vi "test_DL950_temperture.vi"() -> ()   [LabVIEW 2019]
uses:
  76b787d9-b2a3-4b08-af22-58dfa6f6235b.vi
  <instrlib>/Yokogawa DL950 Series/Public/Configure/Configure Module (Voltage).vi
  <instrlib>/Yokogawa DL950 Series/Public/Configure/Configure Module (Temperature).vi
  <instrlib>/Yokogawa DL950 Series/Yokogawa DL950 Series.lvlib
  f7627c64-1743-497c-a0ce-b64357051876.vi
panel:
  out "Waveform Data":waveform(dbl)[](graph)
  in  "Boolean 2":bool
  out "Array":dbl[](array[numeric])
  out "Waveform Chart":T1(graph)
  in  "write buffer":string=":CHANnel3:TEMPerature?"
  out "read buffer":string
  in  "Boolean":bool
  out "time":u32
  in  "정지":bool
  out "error out":errorcluster
  in  "visa":refnum<visa-resource-name>
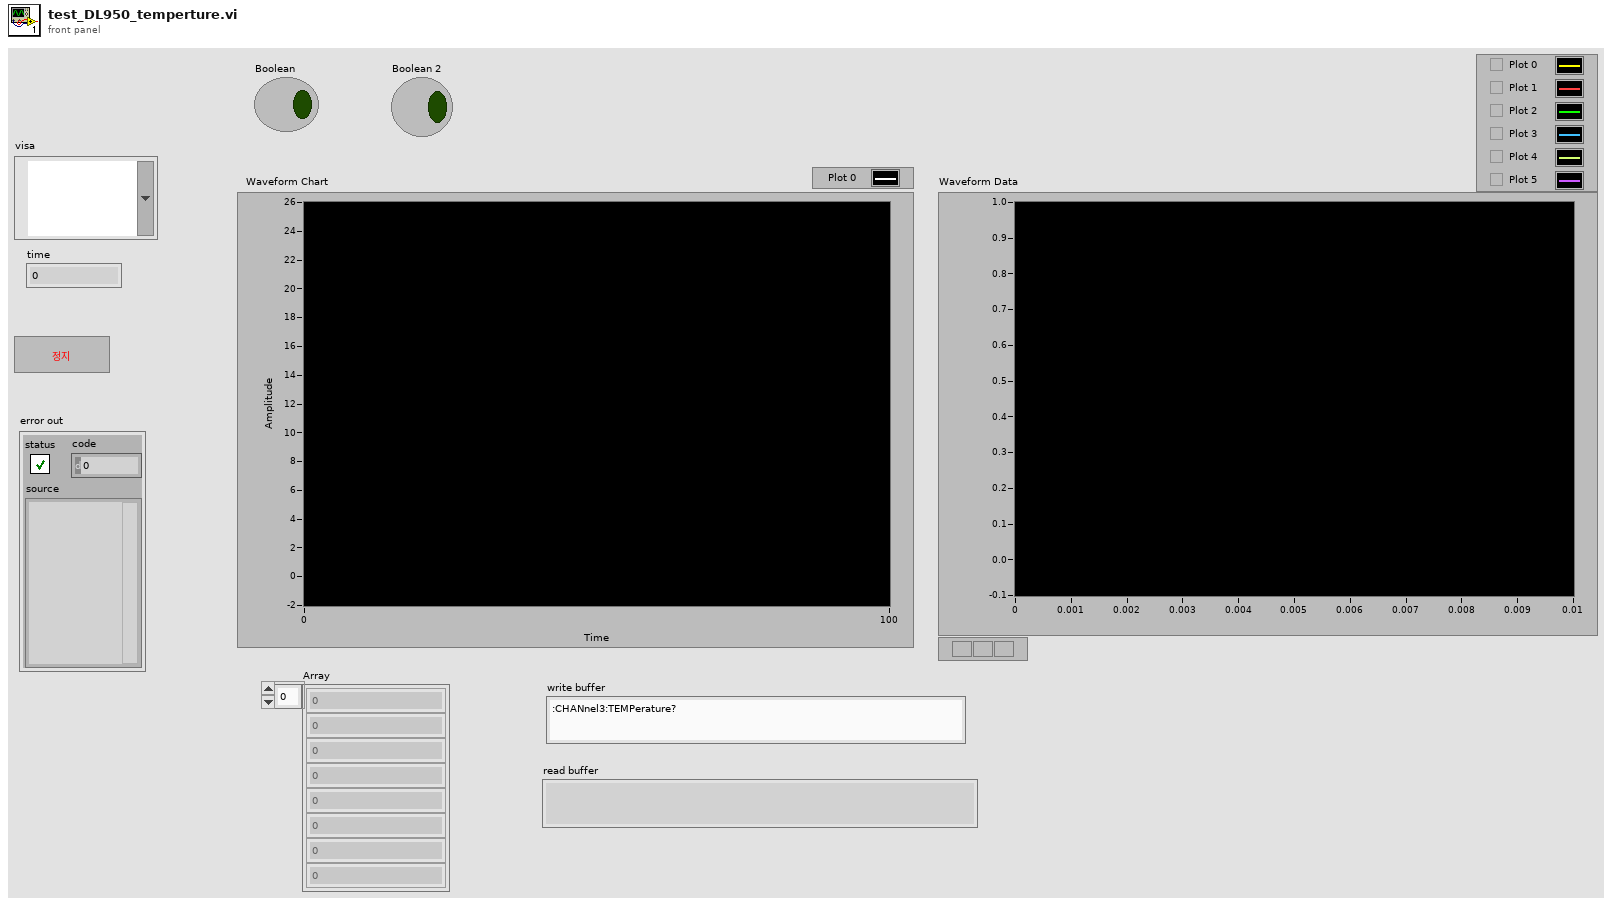
[diagram p1: front panel]
types:
  T1 = cluster{"[0]":dbl, "[1]":dbl, "[2]":dbl, "[3]":dbl, "[4]":dbl, "[5]":dbl, "[6]":dbl, "[7]":dbl, "[8]":dbl}
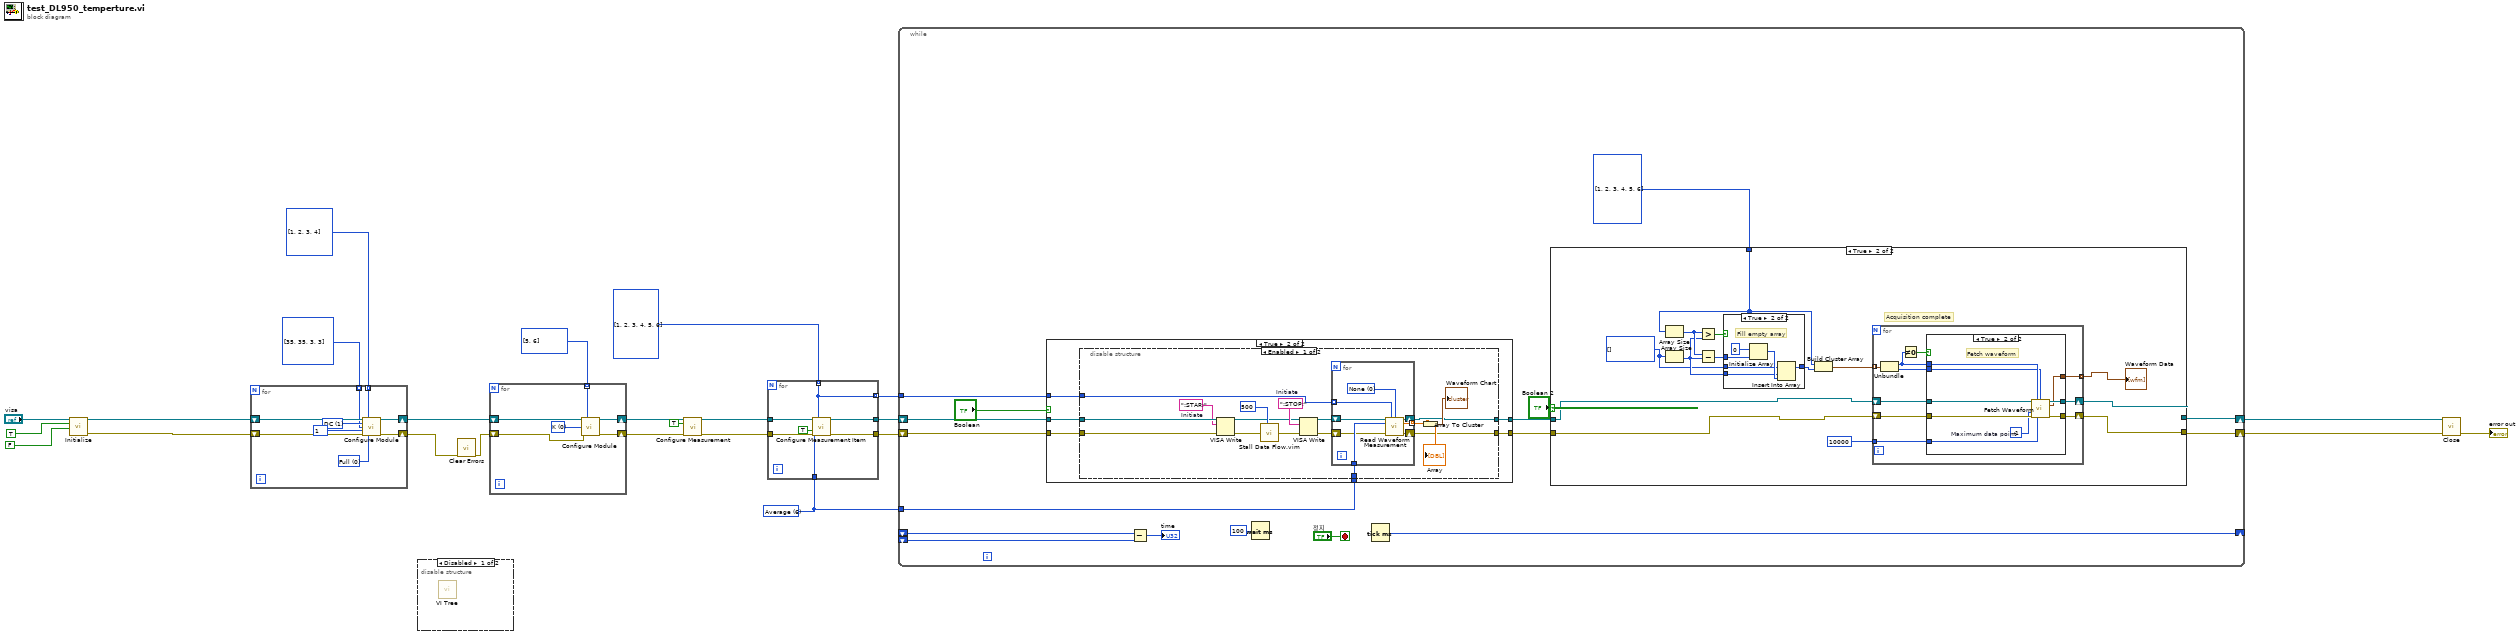
[diagram p0: block diagram]
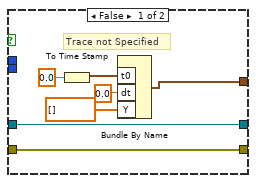
[diagram p4: hidden frame]
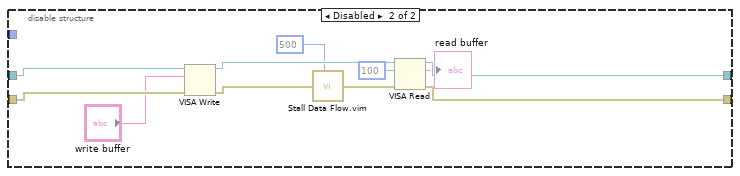
[diagram p7: hidden frame]
diagram:
  w8 = i32[] [35, 35, 3, 3] items=["1:1", "2:1", "5:1", "10:1", "20:1", "50:1", "100:1", "200:1", "500:1", "1000:1", "2000:1", "5000:1", "10k:1", "20k:1", "50k:1", "0.1A:1V", "0.2A:1V", "0.5A:1V", "1A:1V", "2A:1V", "5A:1V", "10A:1V", "20A:1V", "50A:1V", "100A:1V", "200A:1V", "250A:1V", "400A:1V", "500A:1V", "1kA:1V", "2kA:1V", "5kA:1V", "10kA:1V", "20kA:1V", "50kA:1V", "NoSet"]
  w9 = u16[] [1, 2, 3, 4] items=["", "CH1", "CH2", "CH3", "CH4", "CH5", "CH6", "CH7", "CH8", "CH9", "CH10", "CH11", "CH12", "CH13", "CH14", "CH15", "CH16"]
  w12 = u16[] [5, 6] items=["", "CH1", "CH2", "CH3", "CH4", "CH5", "CH6", "CH7", "CH8", "CH9", "CH10", "CH11", "CH12", "CH13", "CH14", "CH15", "CH16"]
  w13 = i32[] [1, 2, 3, 4, 5, 6] items=["", "CH1", "CH2", "CH3", "CH4", "CH5", "CH6", "CH7", "CH8", "CH9", "CH10", "CH11", "CH12", "CH13", "CH14", "CH15", "CH16", "RMATH1", "RMATH2", "RMATH3", "RMATH4", "RMATH5", "RMATH6", "RMATH7", "RMATH8", "RMATH9", "RMATH10", "RMATH11", "RMATH12", "RMATH13", "RMATH14", "RMATH15", "RMATH16", "MATH1", "MATH2", "MATH3", "MATH4", "MATH5", "MATH6", "MATH7", "MATH8"]
  w16 = 6 items=["Peak to Peak", "Amplitude", "Max", "Min", "High", "Low", "Average", "Middle", "Rms", "Standard Deviation", "+Overshoot", "-Overshoot", "Rise", "Fall", "Frequency", "Period", "+Width", "-Width", "Duty Cycle", "Pulse Count", "Burst1 Width", "Burst2 Width", "Average Frequency", "Average Period", "Int1TY", "Int2TY"] ("Measurement Item (0: Peak to Peak)")
  n1 = call <instrlib>:"Initialize.vi"("Reset (True)"=FALSE, "ID Query (True)"=TRUE, "VISA resource name"="visa") -> ("error out"=w1:errorcluster, "VISA resource name out"=w2:refnum<visa-resource-name>)  [unwired: 7 in]
  n2 = for {
    shift-right: [w31] -> w14
    shift-left: w2 -> [w33]
    shift-right: [w30] -> w11
    shift-left: w1 -> [w32]
    tunnel: w9 -> [w26] mode=indexing
    tunnel: w8 -> [w25] mode=indexing
    w28 = 12 items=["0.1m", "0.2m", "0.5m", "1m", "2m", "5m", "10m", "20m", "50m", "100m", "200m", "500m", "1", "2", "4", "5", "8", "10", "20", "40", "50", "80", "100", "200", "400", "500", "800", "1k", "2k", "4k", "5k", "8k", "10k", "20k", "25k", "50k", "100k", "250k", "500k", "1000k"] ("Vertical Division (20: 50)")
    w27 = 0 items=["Full", "Auto", "0.1Hz", "1Hz", "2Hz", "8Hz", "30Hz", "40Hz", "400Hz", "500Hz", "4kHz", "5kHz", "10kHz", "20kHz", "40kHz", "50kHz", "80kHz", "160kHz", "320kHz", "400kHz", "500kHz", "640kHz", "1.28MHz", "2MHz", "2.56MHz", "5MHz"] ("Bandwidth (0: Full)")
    w29 = 1 items=["AC", "DC", "Ground", "AC-RMS", "DC-RMS"] ("Vertical Coupling (1: DC)")
    n3 = call-poly <instrlib>:"Configure Module.vi"("VISA resource name"=w33, "Channel (1: CH1)"=w26, "Vertical Coupling (1: DC)"=w29, "Probe Attenuation (3: 10:1)"=w25, "Vertical Division (20: 50)"=w28, "error in (no error)"=w32, "Bandwidth (0: Full)"=w27) -> ("VISA resource name out"=w31:refnum<visa-resource-name>, "error out"=w30:errorcluster)  [unwired: 7 in]
  }
  n4 = disable-structure shown="Disabled" {
    frame Disabled {
      n5 = call <instrlib>:"VI Tree.vi"() -> ()  [unwired: 12 in]
    }
    frame Enabled {
    }
  }
  n6 = call <vilib>:"Clear Errors.vi"("error in (no error)"=w11) -> ("error out"=w10:errorcluster)  [unwired: 5 in, 1 out]
  n7 = for {
    shift-right: [w35] -> w5
    shift-left: w10 -> [w38]
    shift-right: [w36] -> w7
    shift-left: w14 -> [w37]
    tunnel: w12 -> [w34] mode=indexing
    w39 = 0 items=["K", "E", "J", "T", "L", "U", "N", "R", "S", "B", "W", "Au7fe"] ("Thermocouple Type (0: K)")
    n8 = call-poly <instrlib>:"Configure Module.vi"("VISA resource name"=w37, "Channel (1: CH1)"=w34, "Thermocouple Type (0: K)"=w39, "error in (no error)"=w38) -> ("VISA resource name out"=w36:refnum<visa-resource-name>, "error out"=w35:errorcluster)  [unwired: 10 in]
  }
  n9 = call <instrlib>:"Configure Measurement.vi"("VISA resource name"=w7, "Enable Measurement (True)"=TRUE, "error in (no error)"=w5) -> ("VISA resource name out"=w6:refnum<visa-resource-name>, "error out"=w4:errorcluster)  [unwired: 11 in]
  n10 = for {
    tunnel: [w46] -> w18
    tunnel: [w45] -> w17
    tunnel: w16 -> [w43]
    tunnel: [w40] -> w15 mode=indexing
    tunnel: w6 -> [w42]
    tunnel: w4 -> [w41]
    tunnel: w13 -> [w40] mode=indexing
    n11 = call <instrlib>:"Configure Measurement Item.vi"("VISA resource name"=w42, "Source (1: CH1)"=w40, "Measurement Item (0: Peak to Peak)"=w43, "Enable Measurement Item (False)"=TRUE, "error in (no error)"=w41) -> ("VISA resource name out"=w46:refnum<visa-resource-name>, "error out"=w45:errorcluster)  [unwired: 9 in]
  }
  n12 = while {
    shift-right: [w49] -> w20
    shift-left: w18 -> [w58]
    shift-right: [w48] -> w19
    shift-left: w17 -> [w57]
    shift-right: [w62] -> _
    shift-left: _ -> [w61]
    shift-left: _ -> [w60]
    tunnel: w16 -> [w56]
    tunnel: w15 -> [w53]
    stop <- "정지" stop-if-true
    w47 = u16[] [1, 2, 3, 4, 5, 6] items=["None", "CH1", "CH2", "CH3", "CH4", "CH5", "CH6", "CH7", "CH8", "CH9", "CH10", "CH11", "CH12", "CH13", "CH14", "CH15", "CH16", "MATH1", "MATH2", "MATH3", "MATH4", "MATH5", "MATH6", "MATH7", "MATH8", "EVENT"] ("Source (1: CH1)")
    n13 = case shown="True" "Boolean" {
      tunnel: w58 -> [w114 w120]
      tunnel: w57 -> [w113 w119]
      tunnel: [w114 w118] -> w51
      tunnel: [w113 w117] -> w50
      tunnel: w56 -> [_ w116]
      tunnel: w53 -> [_ w115]
      frame False {
      }
      frame True {
        n14 = disable-structure shown="Enabled" {
          disable-tunnel: w120 -> [w136 w155]
          disable-tunnel: w119 -> [w135 w154]
          disable-tunnel: [w122 w151] -> w118
          disable-tunnel: [w121 w150] -> w117
          disable-tunnel: w116 -> [w134 _]
          disable-tunnel: w115 -> [w125 _]
          frame Enabled {
            w130 = ":STOP;"  # Initiate
            w131 = ":STAR;"  # Initiate
            n15 = VISA Write ("VISA書き込み")(VISA resource name=w136, write buffer=w131, error in (no error)=w135) -> (VISA resource name out=w126:refnum<visa-resource-name>, error out=w129:errorcluster)  [unwired: 1 out]
            n16 = call "Stall Data Flow.vim"("value in"=w129, "milliseconds to wait"=u32 500 ("dt")) -> ("value out"=w128:errorcluster)  [unwired: 1 out]
            n17 = VISA Write ("VISA書き込み")(VISA resource name=w126, write buffer=w130, error in (no error)=w128) -> (VISA resource name out=w133:refnum<visa-resource-name>, error out=w132:errorcluster)  [unwired: 1 out]
            n18 = for {
              tunnel: w134 -> [w142]
              tunnel: [w138] -> w124 mode=indexing
              tunnel: w125 -> [w137] mode=indexing
              shift-right: [w144] -> w122
              shift-left: w133 -> [w140]
              shift-right: [w143] -> w121
              shift-left: w132 -> [w139]
              w141 = i16 0 items=["None", "SCH1", "SCH2", "SCH3", "SCH4", "SCH5", "SCH6", "SCH7", "SCH8", "SCH9", "SCH10", "SCH11", "SCH12", "SCH13", "SCH14", "SCH15", "SCH16", "SCH17", "SCH18", "SCH19", "SCH20", "SCH21", "SCH22", "SCH23", "SCH24", "SCH25", "SCH26", "SCH27", "SCH28", "SCH29", "SCH30", "SCH31", "SCH32", "SCH33", "SCH34", "SCH35", "SCH36", "SCH37", "SCH38", "SCH39", "SCH40", "SCH41", "SCH42", "SCH43", "SCH44", "SCH45", "SCH46", "SCH47", "SCH48", "SCH49", "SCH50", "SCH51", "SCH52", "SCH53", "SCH54", "SCH55", "SCH56", "SCH57", "SCH58", "SCH59", "SCH60", "SCH61", "SCH62", "SCH63", "SCH64"] ("Sub Channel (0: None)")
              n19 = call <instrlib>:"Read Waveform Measurement.vi"("VISA resource name"=w140, "Source (1: CH1)"=w137, "Sub Channel (0: None)"=w141, "Measurement Item (0: Peak to Peak)"=w142, "error in (no error)"=w139) -> ("VISA resource name out"=w144:refnum<visa-resource-name>, "Measurement Value"=w138:dbl, "error out"=w143:errorcluster)  [unwired: 8 in]
            }
            "Array" <- w124
            n20 = Array To Cluster(array=w124) -> (cluster=→"Waveform Chart":T1)
          }
          frame Disabled {
            n21 = VISA Write(VISA resource name=w155, write buffer="write buffer", error in (no error)=w154) -> (VISA resource name out=w153:refnum<visa-resource-name>, error out=w152:errorcluster)  [unwired: 1 out]
            n22 = call "Stall Data Flow.vim"("value in"=w152, "milliseconds to wait"=u32 500) -> ("value out"=w149:errorcluster)  [unwired: 1 out]
            n23 = VISA Read(VISA resource name=w153, byte count=u32 100, error in (no error)=w149) -> (VISA resource name out=w151:refnum<visa-resource-name>, read buffer=→"read buffer":string, error out=w150:errorcluster)  [unwired: 1 out]
          }
        }
      }
    }
    n24 = Subtract(x=w61, y=w60) -> (x-y=→"time":u32)
    n25 = Wait (ms)(milliseconds to wait=u32 100) -> ()  [unwired: 1 out]
    n26 = Tick Count (ms)() -> (millisecond timer value=w62:u32)
    n27 = case shown="True" "Boolean 2" {
      tunnel: w51 -> [w65 w67]
      tunnel: w50 -> [w64 w66]
      tunnel: [w65 w70] -> w49
      tunnel: [w64 w69] -> w48
      tunnel: w47 -> [_ w71]
      frame False {
      }
      frame True {
        w75 = u16[] [] items=["None", "SCH1", "SCH2", "SCH3", "SCH4", "SCH5", "SCH6", "SCH7", "SCH8", "SCH9", "SCH10", "SCH11", "SCH12", "SCH13", "SCH14", "SCH15", "SCH16", "SCH17", "SCH18", "SCH19", "SCH20", "SCH21", "SCH22", "SCH23", "SCH24", "SCH25", "SCH26", "SCH27", "SCH28", "SCH29", "SCH30", "SCH31", "SCH32", "SCH33", "SCH34", "SCH35", "SCH36", "SCH37", "SCH38", "SCH39", "SCH40", "SCH41", "SCH42", "SCH43", "SCH44", "SCH45", "SCH46", "SCH47", "SCH48", "SCH49", "SCH50", "SCH51", "SCH52", "SCH53", "SCH54", "SCH55", "SCH56", "SCH57", "SCH58", "SCH59", "SCH60", "SCH61", "SCH62", "SCH63", "SCH64"] ("Sub Channel (0: None)")
        # "Acquisition complete"
        n28 = Array Size ("配列サイズ")(array=w71) -> (size(s)=w78:i32)
        n29 = Array Size ("配列サイズ")(array=w75) -> (size(s)=w76:i32)
        n30 = Greater? ("大きい?")(x=w78, y=w76) -> (0:w79:bool)
        n31 = Subtract ("·")(x=w78, y=w76) -> (x-y=w77:i32)
        n32 = case "ケースストラクチャ" shown="True" w79 {
          tunnel: w77 -> [_ w111]
          tunnel: [w106 w108] -> w74
          tunnel: w76 -> [_ w107]
          tunnel: w75 -> [w106 w109]
          frame False {
          }
          frame True {
            # "Fill empty array"
            n33 = Initialize Array ("zñú»")(i16 0 ("—v‘f"), w111) -> (w110:i16[])
            n34 = Insert Into Array ("”z—ñ—v‘f‘}“ü")(array=w109, index=w107, new element=w110) -> (w108:u16[])
          }
        }
        n35 = Build Cluster Array ("指標 & バンドルクラスタ配列")(w71, w74) -> (w73:cluster{u16, "Sub Channel (None: 0)":u16}[])
        n36 = for "Forループ" {
          tunnel: [w81] -> w68 mode=indexing
          shift-right: [w85] -> w70
          shift-left: w67 -> [w88]
          shift-right: [w84] -> w69
          shift-left: w66 -> [w87]
          tunnel: w73 -> [w89] mode=indexing
          tunnel: u32 10000 ("Timeout (10000 ms)") -> [w80]
          n37 = Unbundle ("バンドル解除")(w89) -> (w82:u16, "Sub Channel (None: 0)"=w86:u16)
          n38 = Not Equal To 0? ("0に等しくない?")(x=w82) -> (x != 0?=w83:bool)
          n39 = case "ケースストラクチャ" shown="True" w83 {
            tunnel: w88 -> [w96 w105]
            tunnel: w87 -> [w95 w104]
            tunnel: w82 -> [_ w99]
            tunnel: w86 -> [_ w98]
            tunnel: [w96 w103] -> w85
            tunnel: [w95 w102] -> w84
            tunnel: [w90 w101] -> w81
            tunnel: w80 -> [_ w100]
            frame False {
              # "Trace not Specified"
              n40 = To Time Stamp(1:0.0) -> (0:w92:timestamp)
              n41 = Bundle By Name ("Build Waveform")("t0"=w92, "dt"=0.0, "Y"=dbl[] []) -> (w90:waveform(dbl))  [unwired: 1 in]
            }
            frame True {
              w97 = -1  # Maximum data point
              # "Fetch waveform"
              n42 = call <instrlib>:"Fetch Waveform.vi"("VISA resource name"=w105, "Source (1: CH1)"=w99, "Sub Channel(0: None)"=w98, "End Point(1000)"=w97, "error in (no error)"=w104, "Timeout (10000 ms)"=w100) -> ("VISA resource name out"=w103:refnum<visa-resource-name>, "Waveform Data"=w101:waveform(dbl), "error out"=w102:errorcluster)  [unwired: 7 in]
            }
          }
        }
        "Waveform Data" <- w68
      }
    }
  }
  n43 = call <instrlib>:"Close.vi"("error in (no error)"=w19, "VISA resource name"=w20) -> ("error out"=→"error out":errorcluster)  [unwired: 9 in]
